vi "generateInternalError.vi"(8 "error in (no error)":errorcluster, 11 "tcpServer in":refnum<class "TcpServer.lvclass">) -> (0 "error out":errorcluster, 3 "tcpServer out":refnum<class "TcpServer.lvclass">)   [LabVIEW 2018]
doc: "Generate an internal error."
uses:
  src/TcpServer/TcpServer.lvclass
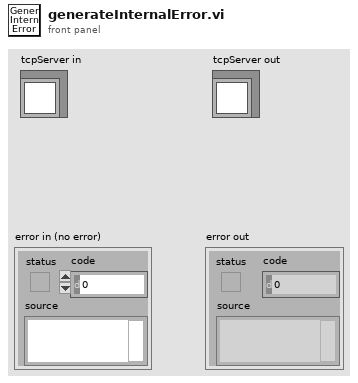
[diagram p1: front panel]
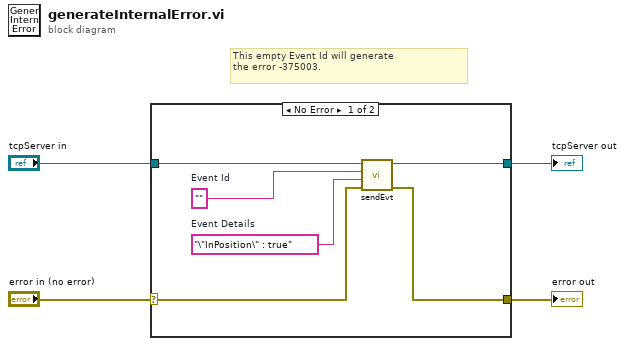
[diagram p0: block diagram]
diagram:
  # "This empty Event Id will generate \nthe error -375003."
  n1 = case shown="No Error" "error in (no error)" {
    selector: "error in (no error)" -> [w6 w11]
    tunnel: "tcpServer in" -> [w10 w12]
    tunnel: [w9 w12] -> w3
    tunnel: [w5 w11] -> w1
    frame No Error {
      w7 = "\"InPosition\" : true"  # Event Details
      w8 = ""  # Event Id
      n2 = call "sendEvt.vi"("error in (no error)"=w6, "Event Details"=w7, "Event Id"=w8, "tcpServer in"=w10) -> ("error out"=w5:errorcluster, "tcpServer out"=w9:refnum<class "TcpServer.lvclass">)  [unwired: 6 in]
    }
    frame Error {
    }
  }
  "tcpServer out" <- w3
  "error out" <- w1
